vi "Pre Launch Init.vi"(11 "Chat Server in":refnum<class "Chat Server.lvclass">) -> (0 "error out":errorcluster, 3 "Chat Server out":refnum<class "Chat Server.lvclass">)   [LabVIEW 2021, in "Chat Server.lvlib" / "Chat Server.lvclass"]
doc: "(<B>Filename</B>: Actor Framework.lvlib:Actor.lvclass:Pre Launch Init.vi)\n\nDefines behavior that occurs after the Launch Nested Actor method is invoked but before the actor's Actor Core method begins running.\n\nBy default, this method does nothing. A descendant class may override it to define behavior."
uses:
  Chat Server.lvclass
  Chat Server.lvclass/Chat Server.ctl
  <vilib>/ActorFramework/Actor/Actor.lvclass
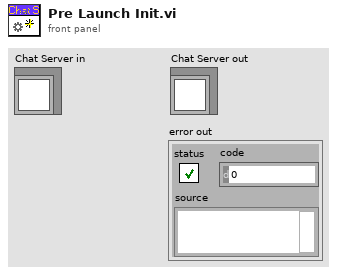
[diagram p1: front panel]
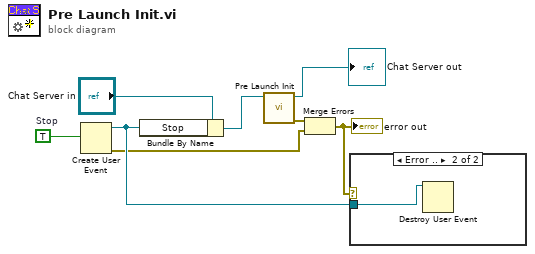
[diagram p0: block diagram]
diagram:
  w7 = TRUE  # Stop
  n1 = Create User Event(user event datatype=w7) -> (user event=w2:refnum<user-event>, error out=w1:errorcluster)  [unwired: 1 in]
  n2 = Bundle By Name(cluster="Chat Server in", "Stop"=w2) -> (w5:refnum<class "Chat Server.lvclass">)
  n3 = call-parent "Pre Launch Init.vi"("Actor in"=w5) -> ("error out"=w4:errorcluster, "Actor out"=→"Chat Server out":refnum<class "Chat Server.lvclass">)  [unwired: 9 in]
  n4 = Merge Errors(w4, w1) -> (w3:errorcluster)
  "error out" <- w3
  n5 = case shown="Error .." w3 {
    tunnel: w2 -> [_ w9]
    frame No Error {
    }
    frame Error {
      n6 = Destroy User Event(user event=w9) -> ()  [unwired: 1 in, 1 out]
    }
  }
